vi "Initialize RaF CD.vi"(8 "error in (no error)":errorcluster, 11 "RaF CD Ref in":T1 format="%.0x") -> (0 "error out":errorcluster, 1 "Aliases Section Ref":T1 format="%.0x", 2 "Routes Section Ref":T1 format="%.0x", 3 "RaF CD Ref out":T1 format="%.0x")   [LabVIEW 2017, in "Switch Scripting.lvlib"]
uses:
  Switch Scripting.lvlib
  <vilib>/NI Veristand/Custom Device API/Custom Device Item Ref.ctl
  Shared/Constants.vi
  <vilib>/NI VeriStand/Custom Device API/Custom Device API.lvlib
  Shared/Switch Shared.lvlib
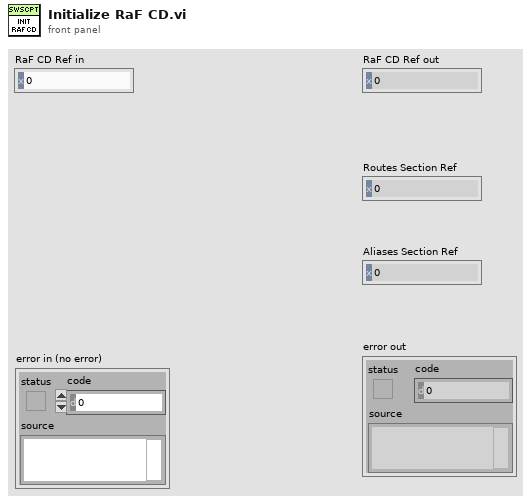
[diagram p1: front panel]
types:
  T1 = typedef "Custom Device API.lvlib/Custom Device Item Ref.ctl" = u64
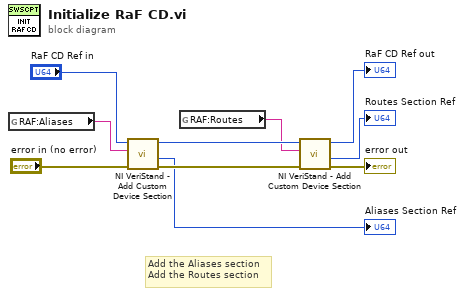
[diagram p0: block diagram]
diagram:
  # "Add the Aliases section\nAdd the Routes section"
  n1 = global read "Constants.vi" "RAF:Aliases"() -> (w2:string)
  n2 = call <vilib>:"NI VeriStand - Add Custom Device Section.vi"("error in (no error)"="error in (no error)", "Section Name"=w2, "Parent Ref in"="RaF CD Ref in") -> ("error out"=w9:errorcluster, "Section Ptr"=→"Aliases Section Ref":T1, "Parent Ref out"=w10:T1)  [unwired: 5 in, 1 out]
  n3 = global read "Constants.vi" "RAF:Routes"() -> (w1:string)
  n4 = call <vilib>:"NI VeriStand - Add Custom Device Section.vi"("error in (no error)"=w9, "Section Name"=w1, "Parent Ref in"=w10) -> ("error out"=→"error out":errorcluster, "Section Ptr"=→"Routes Section Ref":T1, "Parent Ref out"=→"RaF CD Ref out":T1)  [unwired: 5 in, 1 out]
